vi "Read Screen Tap.vi"   [LabVIEW 2011, in "LVH-Leap.lvlib"]
uses:
  LVH-Leap.lvlib
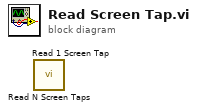
[diagram p0: block diagram]
diagram:
  n1 = call "Read N Screen Taps.vi"() -> ()  [unwired: 8 in, 4 out]
  n2 = call "Read 1 Screen Tap.vi"() -> ()  [unwired: 8 in, 4 out]
